vi "ReadCalibrationData.vi"(0 "reference in":refnum<class "BME280.lvclass">, 5 "error in (no error)":errorcluster, 6 "LINX Resource":T2={"IO"=enum."Remote", "Interface"=enum."Serial", "LINX Device Config"={"Interface"=enum."Serial", "COM Port"="COM13", "TCP Configuration"={"IP Address"="", "Port"=0}, "Device Family"=1, "Device ID"=1, "Device Name"="myRIO-1900", "TCP Ref"=refnum, "Channels"={"DI"=[0, 1, 2, 3, 4, 5, 6, 7, 8, 9, 10, 11, 12, 13, 14, 15, 16, 17, 18, 19, 20, 21, 22, 23, 24, 25, 26, 27, 28, 29, 30, 31, 32, 33, 34, 35, 36, 37, 38, 39, 40, 41, 42, 43, 44, 45, 46], "DO"=[0, 1, 2, 3, 4, 5, 6, 7, 8, 9, 10, 11, 12, 13, 14, 15, 16, 17, 18, 19, 20, 21, 22, 23, 24, 25, 26, 27, 28, 29, 30, 31, 32, 33, 34, 35, 36, 37, 38, 39, 40, 41, 42, 43, 44, 45, 46], "AI"=[0, 1, 2, 3, 4, 5, 6, 7, 8, 9, 10, 11], "AO"=[], "PWM"=[3, 5, 6, 9, 10], "QE"=[], "UART"=[0, 1], "I2C 2"=[0], "SPI"=[0], "CAN"=[], "Servo"=[], "AI Ref (V)"=0.0, "AI Resolution (Bits)"=0, "AO Ref (V)"=0.0, "AO Resolution (Bits)"=0}}}, 8 "I2C Channel (0)":u8=1) -> (12 "LINX Resource":T2={"IO"=enum."Remote", "Interface"=enum."Serial", "LINX Device Config"={"Interface"=enum."Serial", "COM Port"="COM13", "TCP Configuration"={"IP Address"="", "Port"=0}, "Device Family"=1, "Device ID"=1, "Device Name"="myRIO-1900", "TCP Ref"=refnum, "Channels"={"DI"=[0, 1, 2, 3, 4, 5, 6, 7, 8, 9, 10, 11, 12, 13, 14, 15, 16, 17, 18, 19, 20, 21, 22, 23, 24, 25, 26, 27, 28, 29, 30, 31, 32, 33, 34, 35, 36, 37, 38, 39, 40, 41, 42, 43, 44, 45, 46], "DO"=[0, 1, 2, 3, 4, 5, 6, 7, 8, 9, 10, 11, 12, 13, 14, 15, 16, 17, 18, 19, 20, 21, 22, 23, 24, 25, 26, 27, 28, 29, 30, 31, 32, 33, 34, 35, 36, 37, 38, 39, 40, 41, 42, 43, 44, 45, 46], "AI"=[0, 1, 2, 3, 4, 5, 6, 7, 8, 9, 10, 11], "AO"=[], "PWM"=[3, 5, 6, 9, 10], "QE"=[], "UART"=[0, 1], "I2C 2"=[0], "SPI"=[0], "CAN"=[], "Servo"=[], "AI Ref (V)"=0.0, "AI Resolution (Bits)"=0, "AO Ref (V)"=0.0, "AO Resolution (Bits)"=0}}}, 14 "reference out":refnum<class "BME280.lvclass">, 16 "TrimmingParameters":T1, 19 "error out":errorcluster)   [LabVIEW 2014, in "BME280.lvclass"]
uses:
  BME280.lvclass
  <vilib>/MakerHub/LINX/Private/Type Defs/LINX Ref.ctl
  <vilib>/MakerHub/LINX/Private/Type Defs/Platform.ctl
  <vilib>/MakerHub/LINX/Private/Type Defs/Interface.ctl
  <vilib>/MakerHub/LINX/Private/Device/Type Defs/LINX Device Config.ctl
  <vilib>/MakerHub/LINX/Private/Device/Type Defs/TCP Config.ctl
  <vilib>/MakerHub/LINX/Private/Device/Type Defs/Channels.ctl
  TrimmingParameters.ctl
  <vilib>/MakerHub/LINX/Private/Local IO/LinxI2cWrite.vi
  <vilib>/MakerHub/LINX/Public/Utilities/Check Channel.vi
  <vilib>/MakerHub/LINX/Private/Local IO/Handle Errors.vi
  <vilib>/MakerHub/LINX/Private/Utilties/Generate Error.vi
  <vilib>/MakerHub/LINX/LMH-LINX.lvlib
  <vilib>/MakerHub/LINX/Private/Device/Device.lvlib
panel:
  out "Data 3":u8[](array[numeric])
  out "Data 2":u8[](array[numeric])
  out "Data":u8[](array[numeric])
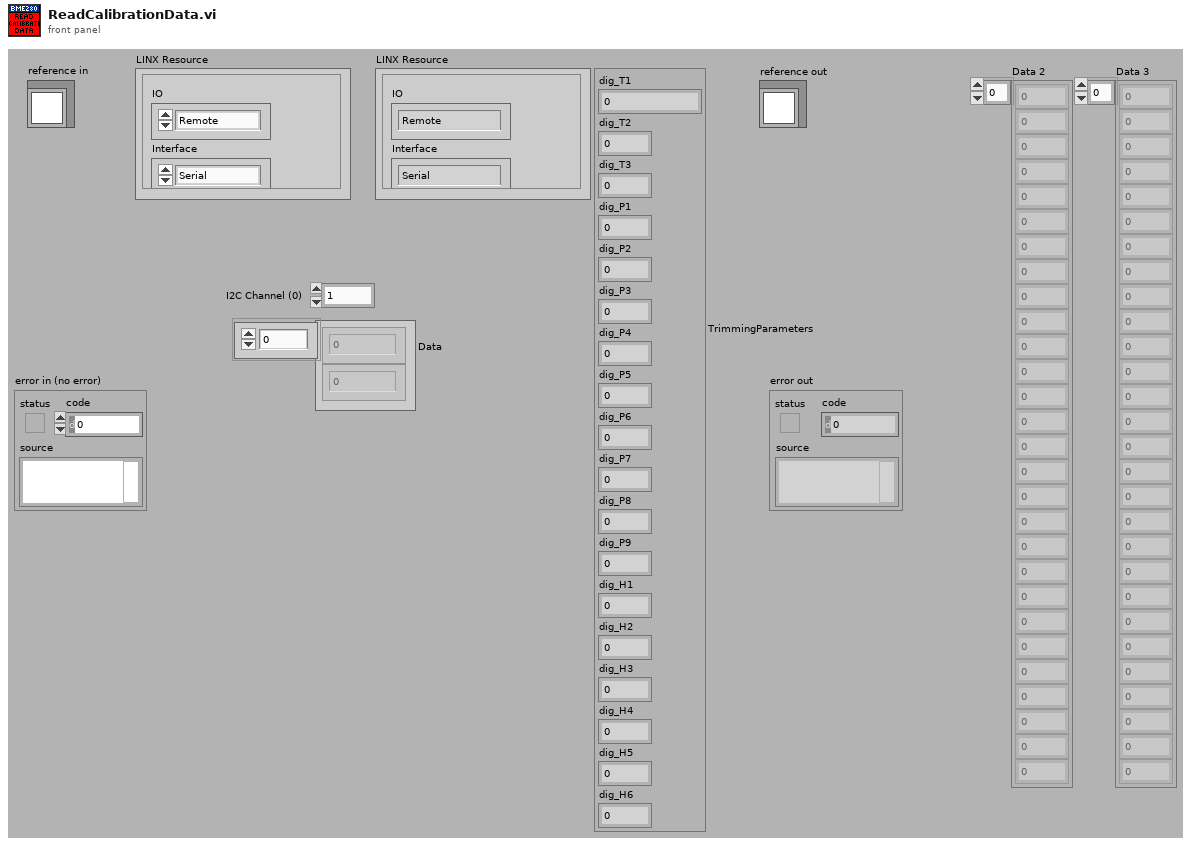
[diagram p1: front panel]
types:
  T1 = typedef "BME280.lvclass/TrimmingParameters.ctl" = cluster{"dig_T1":u16, "dig_T2":i16, "dig_T3":i16, "dig_P1":u16, "dig_P2":i16, "dig_P3":i16, "dig_P4":i16, "dig_P5":i16, "dig_P6":i16, "dig_P7":i16, "dig_P8":i16, "dig_P9":i16, "dig_H1":u8, "dig_H2":i16, "dig_H3":u8, "dig_H4":i16, "dig_H5":i16, "dig_H6":i8}
  T2 = typedef "LMH-LINX.lvlib/LINX Ref.ctl" = cluster{"IO":T3, "Interface":T4, "LINX Device Config":T5}
  T3 = typedef "LMH-LINX.lvlib/Platform.ctl" = enum16{"Remote", "Local"}
  T4 = typedef "LMH-LINX.lvlib/Interface.ctl" = enum16{"Serial", "TCP"}
  T5 = typedef "LMH-LINX.lvlib/Device.lvlib/LINX Device Config.ctl" = cluster{"Interface":T4, "COM Port":refnum<visa-resource-name>, "TCP Configuration":T6, "Device Family":u8, "Device ID":u8, "Device Name":string, "TCP Ref":refnum<k5>, "Channels":T7}
  T6 = typedef "LMH-LINX.lvlib/Device.lvlib/TCP Config.ctl" = cluster{"IP Address":string, "Port":u16}
  T7 = typedef "LMH-LINX.lvlib/Channels.ctl" = cluster{"DI":u8[], "DO":u8[], "AI":u8[], "AO":u8[], "PWM":u8[], "QE":u8[], "UART":u8[], "I2C 2":u8[], "SPI":u8[], "CAN":u8[], "Servo":u8[], "AI Ref (V)":dbl, "AI Resolution (Bits)":u8, "AO Ref (V)":dbl, "AO Resolution (Bits)":u8}
  T8 = typedef "BME280.lvclass/ObjectAttributes.ctl" = cluster{"I2C Slave Address":u8, "TrimmingParameters":T1, "t_fine":i32}
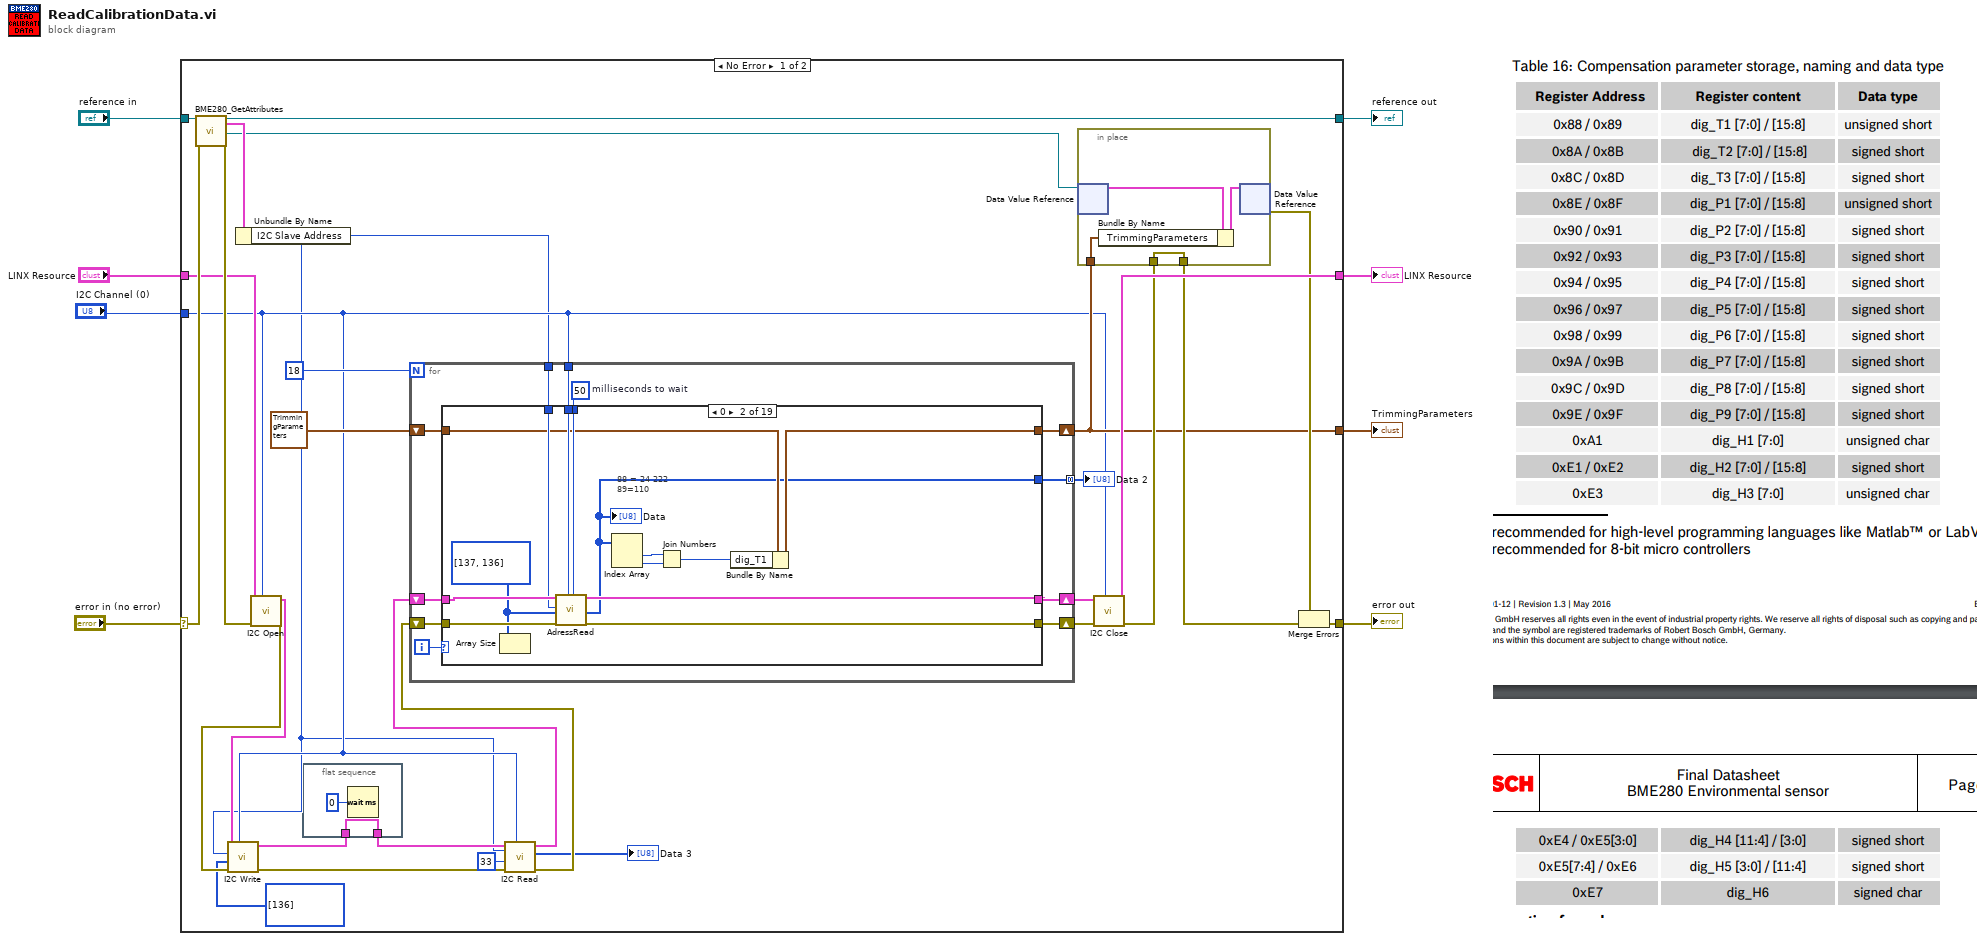
[diagram p0: block diagram]
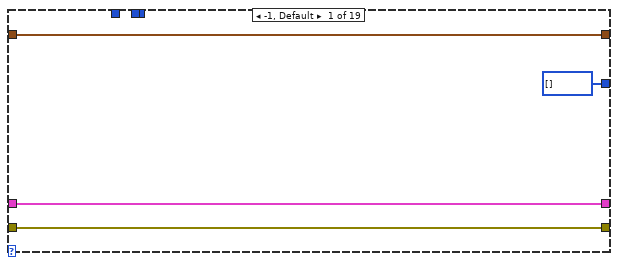
[diagram p2: hidden frame]
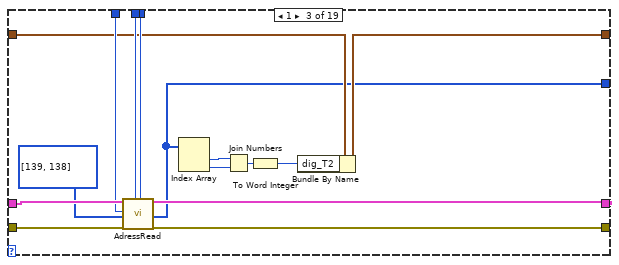
[diagram p3: hidden frame]
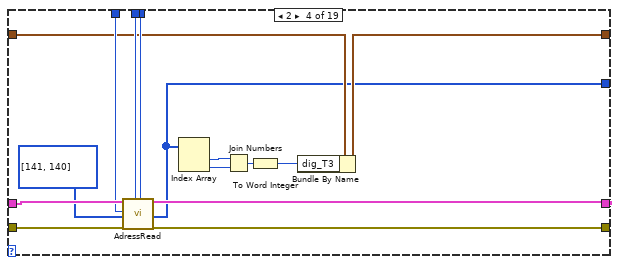
[diagram p4: hidden frame]
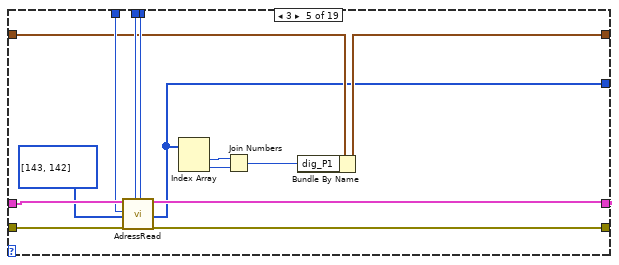
[diagram p5: hidden frame]
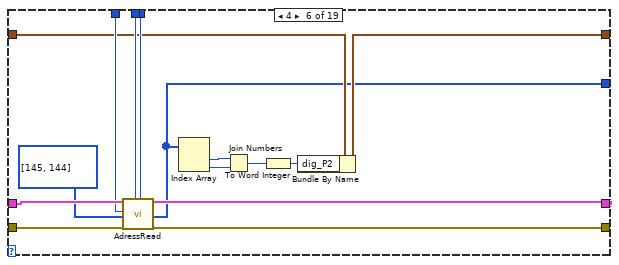
[diagram p6: hidden frame]
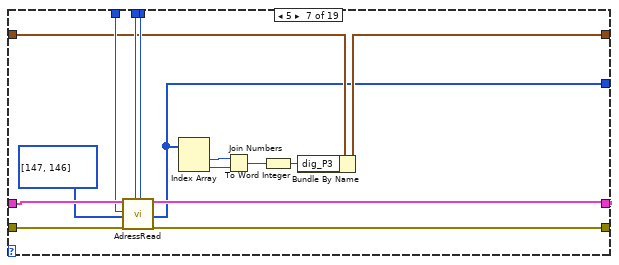
[diagram p7: hidden frame]
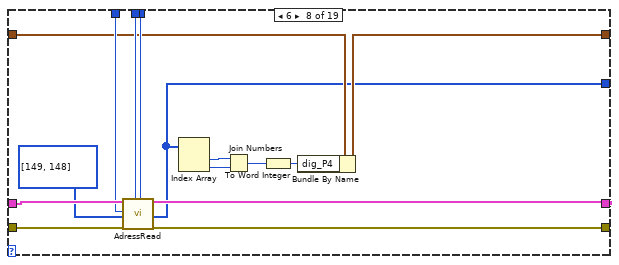
[diagram p8: hidden frame]
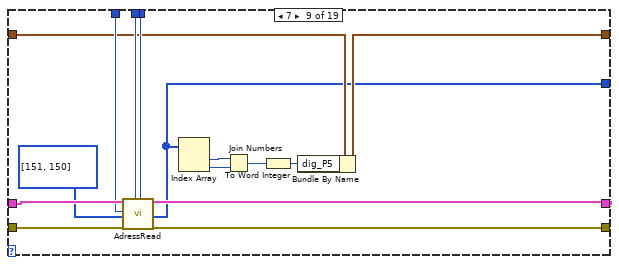
[diagram p9: hidden frame]
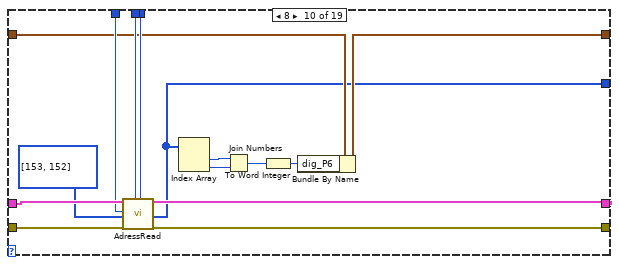
[diagram p10: hidden frame]
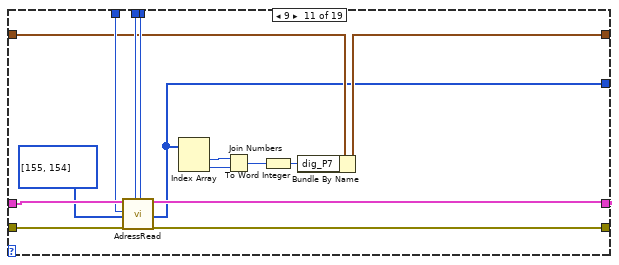
[diagram p11: hidden frame]
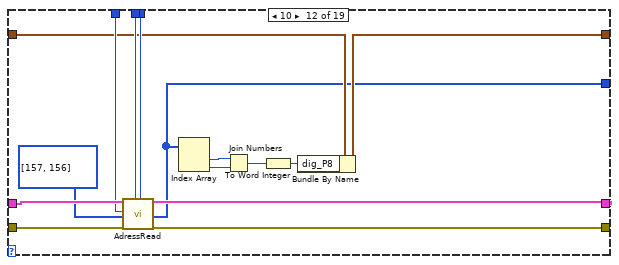
[diagram p12: hidden frame]
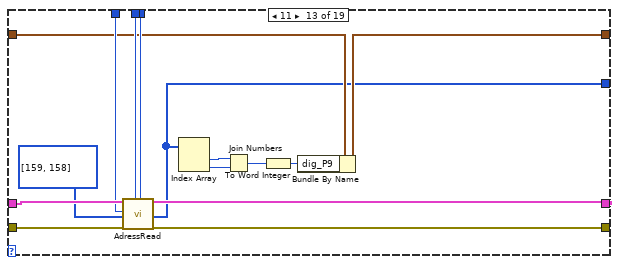
[diagram p13: hidden frame]
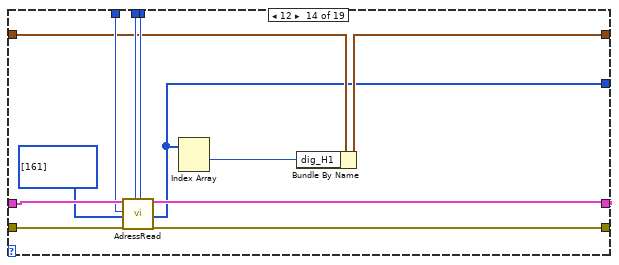
[diagram p14: hidden frame]
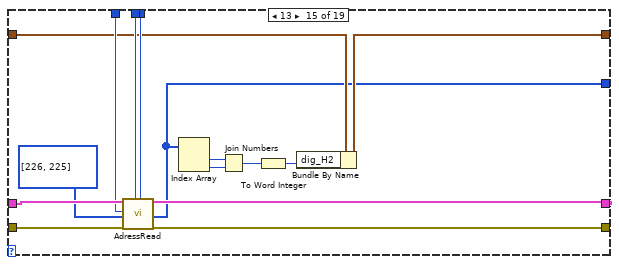
[diagram p15: hidden frame]
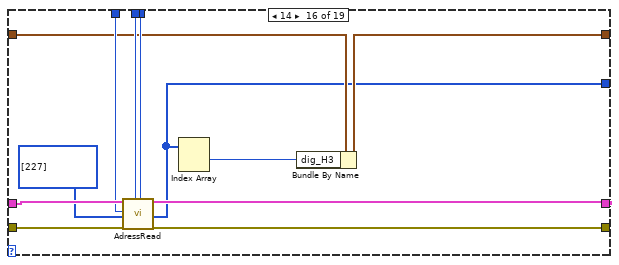
[diagram p16: hidden frame]
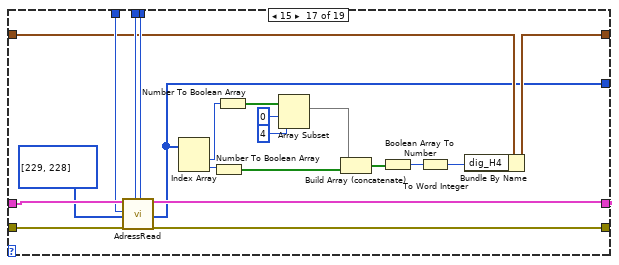
[diagram p17: hidden frame]
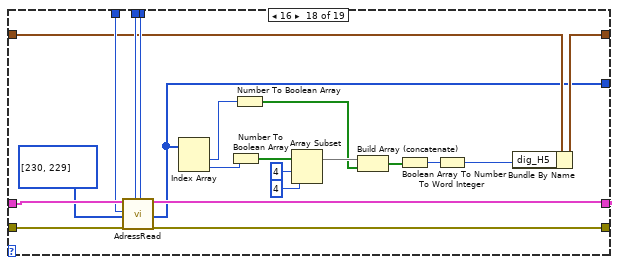
[diagram p18: hidden frame]
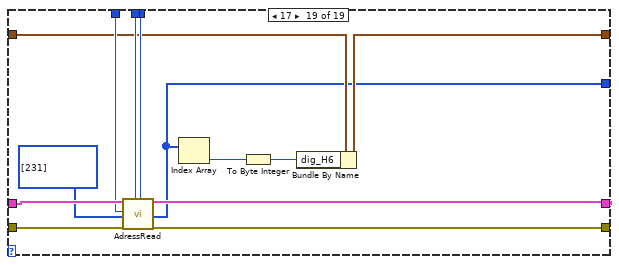
[diagram p19: hidden frame]
diagram:
  n1 = case shown="No Error" "error in (no error)" {
    selector: "error in (no error)" -> [w38 w334]
    tunnel: [w24 w334] -> w7
    tunnel: [w36 w333] -> w5
    tunnel: "reference in" -> [w37 w333]
    tunnel: "LINX Resource" -> [w34 w332]
    tunnel: [w33 w332] -> w3
    tunnel: "I2C Channel (0)" -> [w13 _]
    tunnel: [w22 _] -> w1
    frame No Error {
      n2 = call "BME280_GetAttributes.vi"("reference in"=w37, "error in (no error)"=w38) -> ("reference out"=w36:refnum<class "BME280.lvclass">, "Data"=w32:T8, "DataRef"=w26:refnum<data-value>, "error out"=w35:errorcluster)  [unwired: 14 in]
      n3 = Unbundle By Name(w32) -> ("I2C Slave Address"=w12:u8)
      n4 = call <vilib>:"I2C Open.vi"("I2C Channel (0)"=w13, "Error In"=w35, "LINX Resource"=w34) -> ("Error Out"=w15:errorcluster, "LINX Resource"=w17:T2)  [unwired: 7 in]
      n5 = call <vilib>:"I2C Write.vi"("I2C Channel"=w13, "Error In"=w15, "Data"=u8[] [136] ("Adress"), "I2C Slave Address (0)"=w12, "LINX Resource"=w17) -> ("Error Out"=w18:errorcluster, "LINX Resource"=w19:T2)  [unwired: 5 in]
      n6 = flat-sequence {
        tunnel: [w40] -> w20
        tunnel: w19 -> [w40]
        frame #0 {
          n7 = Wait (ms)(milliseconds to wait=u32 0) -> ()  [unwired: 1 out]
        }
      }
      n8 = call <vilib>:"I2C Read.vi"("I2C Channel"=w13, "Error In"=w18, "Bytes To Read"=u8 33, "I2C Slave Address (0)"=w12, "LINX Resource"=w20) -> ("Error Out"=w14:errorcluster, "Data"=→"Data 3":u8[], "LINX Resource"=w16:T2)  [unwired: 4 in]
      n9 = for {
        N: 18 -> [_]
        shift-right: [w50] -> w31
        shift-left: w16 -> [w51]
        shift-right: [w48] -> w30
        shift-left: w14 -> [w49]
        shift-right: [w44] -> w22
        shift-left: T1 {"dig_T1"=0, "dig_T2"=0, "dig_T3"=0, "dig_P1"=0, "dig_P2"=0, "dig_P3"=0, "dig_P4"=0, "dig_P5"=0, "dig_P6"=0, "dig_P7"=0, "dig_P8"=0, "dig_P9"=0, "dig_H1"=0, "dig_H2"=0, "dig_H3"=0, "dig_H4"=0, "dig_H5"=0, "dig_H6"=0} ("TrimmingParameters") -> [w45]
        tunnel: w12 -> [w43]
        tunnel: w13 -> [w42]
        tunnel: [w41] -> w21 mode=concatenating
        i -> [w46]
        w47 = u32 50  # milliseconds to wait
        n10 = case shown="0" w46 {
          tunnel: w51 -> [w55 w66 w81 w96 w110 w125 w140 w155 w170 w185 w200 w215 w230 w242 w257 w269 w290 w311 w324]
          tunnel: [w55 w69 w84 w99 w113 w128 w143 w158 w173 w188 w203 w218 w233 w245 w260 w272 w293 w314 w327] -> w50
          tunnel: w49 -> [w54 w68 w83 w98 w112 w127 w142 w157 w172 w187 w202 w217 w232 w244 w259 w271 w292 w313 w326]
          tunnel: [w54 w67 w82 w97 w111 w126 w141 w156 w171 w186 w201 w216 w231 w243 w258 w270 w291 w312 w325] -> w48
          tunnel: w47 -> [_ w65 w79 w94 w108 w123 w138 w153 w168 w183 w198 w213 w228 w240 w255 w267 w288 w309 w322]
          tunnel: w45 -> [w53 w60 w74 w89 w103 w118 w133 w148 w163 w178 w193 w208 w223 w237 w252 w264 w285 w306 w319]
          tunnel: [w53 w59 w73 w88 w102 w117 w132 w147 w162 w177 w192 w207 w222 w236 w251 w263 w284 w305 w318] -> w44
          tunnel: w43 -> [_ w63 w77 w92 w106 w121 w136 w151 w166 w181 w196 w211 w226 w238 w253 w265 w286 w307 w320]
          tunnel: w42 -> [_ w64 w78 w93 w107 w122 w137 w152 w167 w182 w197 w212 w227 w239 w254 w266 w287 w308 w321]
          tunnel: [u8[] [] ("Data") w56 w70 w85 w100 w114 w129 w144 w159 w174 w189 w204 w219 w234 w246 w261 w273 w294 w315] -> w41
          frame -1, Default {
          }
          frame 0 {
            w57 = u8[] [137, 136] ("Adress")
            # "88 = 24 222\n89=110"
            n11 = Array Size(array=w57) -> ()  [unwired: 1 out]
            n12 = call "AdressRead.vi"("LINX Resource in"=w66, "I2C Slave Address"=w63, "Adress"=w57, "error in (no error)"=w68, "I2C Channel"=w64, "milliseconds to wait"=w65) -> ("LINX Resource out"=w69:T2, "Data"=w56:u8[], "error out"=w67:errorcluster)  [unwired: 11 in]
            "Data" <- w56
            n13 = Index Array(array=w56) -> (element #1=w62:u8, element #2=w61:u8)  [unwired: 2 in]
            n14 = Join Numbers(hi=w62, lo=w61) -> ((hi.lo)=w58:u16)
            n15 = Bundle By Name(cluster=w60, "dig_T1"=w58) -> (w59:T1)
          }
          frame 1 {
            n16 = call "AdressRead.vi"("LINX Resource in"=w81, "I2C Slave Address"=w77, "Adress"=u8[] [139, 138], "error in (no error)"=w83, "I2C Channel"=w78, "milliseconds to wait"=w79) -> ("LINX Resource out"=w84:T2, "Data"=w70:u8[], "error out"=w82:errorcluster)  [unwired: 11 in]
            n17 = Index Array(array=w70) -> (element #1=w76:u8, element #2=w75:u8)  [unwired: 2 in]
            n18 = Join Numbers(hi=w76, lo=w75) -> ((hi.lo)=w72:u16)
            n19 = To Word Integer(number=w72) -> (16bit integer=w71:i16)
            n20 = Bundle By Name(cluster=w74, "dig_T2"=w71) -> (w73:T1)
          }
          frame 2 {
            n21 = call "AdressRead.vi"("LINX Resource in"=w96, "I2C Slave Address"=w92, "Adress"=u8[] [141, 140], "error in (no error)"=w98, "I2C Channel"=w93, "milliseconds to wait"=w94) -> ("LINX Resource out"=w99:T2, "Data"=w85:u8[], "error out"=w97:errorcluster)  [unwired: 11 in]
            n22 = Index Array(array=w85) -> (element #1=w91:u8, element #2=w90:u8)  [unwired: 2 in]
            n23 = Join Numbers(hi=w91, lo=w90) -> ((hi.lo)=w87:u16)
            n24 = To Word Integer(number=w87) -> (16bit integer=w86:i16)
            n25 = Bundle By Name(cluster=w89, "dig_T3"=w86) -> (w88:T1)
          }
          frame 3 {
            n26 = call "AdressRead.vi"("LINX Resource in"=w110, "I2C Slave Address"=w106, "Adress"=u8[] [143, 142], "error in (no error)"=w112, "I2C Channel"=w107, "milliseconds to wait"=w108) -> ("LINX Resource out"=w113:T2, "Data"=w100:u8[], "error out"=w111:errorcluster)  [unwired: 11 in]
            n27 = Index Array(array=w100) -> (element #1=w105:u8, element #2=w104:u8)  [unwired: 2 in]
            n28 = Join Numbers(hi=w105, lo=w104) -> ((hi.lo)=w101:u16)
            n29 = Bundle By Name(cluster=w103, "dig_P1"=w101) -> (w102:T1)
          }
          frame 4 {
            n30 = call "AdressRead.vi"("LINX Resource in"=w125, "I2C Slave Address"=w121, "Adress"=u8[] [145, 144], "error in (no error)"=w127, "I2C Channel"=w122, "milliseconds to wait"=w123) -> ("LINX Resource out"=w128:T2, "Data"=w114:u8[], "error out"=w126:errorcluster)  [unwired: 11 in]
            n31 = Index Array(array=w114) -> (element #1=w120:u8, element #2=w119:u8)  [unwired: 2 in]
            n32 = Join Numbers(hi=w120, lo=w119) -> ((hi.lo)=w116:u16)
            n33 = To Word Integer(number=w116) -> (16bit integer=w115:i16)
            n34 = Bundle By Name(cluster=w118, "dig_P2"=w115) -> (w117:T1)
          }
          frame 5 {
            n35 = call "AdressRead.vi"("LINX Resource in"=w140, "I2C Slave Address"=w136, "Adress"=u8[] [147, 146], "error in (no error)"=w142, "I2C Channel"=w137, "milliseconds to wait"=w138) -> ("LINX Resource out"=w143:T2, "Data"=w129:u8[], "error out"=w141:errorcluster)  [unwired: 11 in]
            n36 = Index Array(array=w129) -> (element #1=w135:u8, element #2=w134:u8)  [unwired: 2 in]
            n37 = Join Numbers(hi=w135, lo=w134) -> ((hi.lo)=w131:u16)
            n38 = To Word Integer(number=w131) -> (16bit integer=w130:i16)
            n39 = Bundle By Name(cluster=w133, "dig_P3"=w130) -> (w132:T1)
          }
          frame 6 {
            n40 = call "AdressRead.vi"("LINX Resource in"=w155, "I2C Slave Address"=w151, "Adress"=u8[] [149, 148], "error in (no error)"=w157, "I2C Channel"=w152, "milliseconds to wait"=w153) -> ("LINX Resource out"=w158:T2, "Data"=w144:u8[], "error out"=w156:errorcluster)  [unwired: 11 in]
            n41 = Index Array(array=w144) -> (element #1=w150:u8, element #2=w149:u8)  [unwired: 2 in]
            n42 = Join Numbers(hi=w150, lo=w149) -> ((hi.lo)=w146:u16)
            n43 = To Word Integer(number=w146) -> (16bit integer=w145:i16)
            n44 = Bundle By Name(cluster=w148, "dig_P4"=w145) -> (w147:T1)
          }
          frame 7 {
            n45 = call "AdressRead.vi"("LINX Resource in"=w170, "I2C Slave Address"=w166, "Adress"=u8[] [151, 150], "error in (no error)"=w172, "I2C Channel"=w167, "milliseconds to wait"=w168) -> ("LINX Resource out"=w173:T2, "Data"=w159:u8[], "error out"=w171:errorcluster)  [unwired: 11 in]
            n46 = Index Array(array=w159) -> (element #1=w165:u8, element #2=w164:u8)  [unwired: 2 in]
            n47 = Join Numbers(hi=w165, lo=w164) -> ((hi.lo)=w161:u16)
            n48 = To Word Integer(number=w161) -> (16bit integer=w160:i16)
            n49 = Bundle By Name(cluster=w163, "dig_P5"=w160) -> (w162:T1)
          }
          frame 8 {
            n50 = call "AdressRead.vi"("LINX Resource in"=w185, "I2C Slave Address"=w181, "Adress"=u8[] [153, 152], "error in (no error)"=w187, "I2C Channel"=w182, "milliseconds to wait"=w183) -> ("LINX Resource out"=w188:T2, "Data"=w174:u8[], "error out"=w186:errorcluster)  [unwired: 11 in]
            n51 = Index Array(array=w174) -> (element #1=w180:u8, element #2=w179:u8)  [unwired: 2 in]
            n52 = Join Numbers(hi=w180, lo=w179) -> ((hi.lo)=w176:u16)
            n53 = To Word Integer(number=w176) -> (16bit integer=w175:i16)
            n54 = Bundle By Name(cluster=w178, "dig_P6"=w175) -> (w177:T1)
          }
          frame 9 {
            n55 = call "AdressRead.vi"("LINX Resource in"=w200, "I2C Slave Address"=w196, "Adress"=u8[] [155, 154], "error in (no error)"=w202, "I2C Channel"=w197, "milliseconds to wait"=w198) -> ("LINX Resource out"=w203:T2, "Data"=w189:u8[], "error out"=w201:errorcluster)  [unwired: 11 in]
            n56 = Index Array(array=w189) -> (element #1=w195:u8, element #2=w194:u8)  [unwired: 2 in]
            n57 = Join Numbers(hi=w195, lo=w194) -> ((hi.lo)=w191:u16)
            n58 = To Word Integer(number=w191) -> (16bit integer=w190:i16)
            n59 = Bundle By Name(cluster=w193, "dig_P7"=w190) -> (w192:T1)
          }
          frame 10 {
            n60 = call "AdressRead.vi"("LINX Resource in"=w215, "I2C Slave Address"=w211, "Adress"=u8[] [157, 156], "error in (no error)"=w217, "I2C Channel"=w212, "milliseconds to wait"=w213) -> ("LINX Resource out"=w218:T2, "Data"=w204:u8[], "error out"=w216:errorcluster)  [unwired: 11 in]
            n61 = Index Array(array=w204) -> (element #1=w210:u8, element #2=w209:u8)  [unwired: 2 in]
            n62 = Join Numbers(hi=w210, lo=w209) -> ((hi.lo)=w206:u16)
            n63 = To Word Integer(number=w206) -> (16bit integer=w205:i16)
            n64 = Bundle By Name(cluster=w208, "dig_P8"=w205) -> (w207:T1)
          }
          frame 11 {
            n65 = call "AdressRead.vi"("LINX Resource in"=w230, "I2C Slave Address"=w226, "Adress"=u8[] [159, 158], "error in (no error)"=w232, "I2C Channel"=w227, "milliseconds to wait"=w228) -> ("LINX Resource out"=w233:T2, "Data"=w219:u8[], "error out"=w231:errorcluster)  [unwired: 11 in]
            n66 = Index Array(array=w219) -> (element #1=w225:u8, element #2=w224:u8)  [unwired: 2 in]
            n67 = Join Numbers(hi=w225, lo=w224) -> ((hi.lo)=w221:u16)
            n68 = To Word Integer(number=w221) -> (16bit integer=w220:i16)
            n69 = Bundle By Name(cluster=w223, "dig_P9"=w220) -> (w222:T1)
          }
          frame 12 {
            n70 = call "AdressRead.vi"("LINX Resource in"=w242, "I2C Slave Address"=w238, "Adress"=u8[] [161], "error in (no error)"=w244, "I2C Channel"=w239, "milliseconds to wait"=w240) -> ("LINX Resource out"=w245:T2, "Data"=w234:u8[], "error out"=w243:errorcluster)  [unwired: 11 in]
            n71 = Index Array(array=w234) -> (element #1=w235:u8)  [unwired: 2 in, 1 out]
            n72 = Bundle By Name(cluster=w237, "dig_H1"=w235) -> (w236:T1)
          }
          frame 13 {
            n73 = call "AdressRead.vi"("LINX Resource in"=w257, "I2C Slave Address"=w253, "Adress"=u8[] [226, 225], "error in (no error)"=w259, "I2C Channel"=w254, "milliseconds to wait"=w255) -> ("LINX Resource out"=w260:T2, "Data"=w246:u8[], "error out"=w258:errorcluster)  [unwired: 11 in]
            n74 = Index Array(array=w246) -> (element #1=w249:u8, element #2=w248:u8)  [unwired: 2 in]
            n75 = Join Numbers(hi=w249, lo=w248) -> ((hi.lo)=w250:u16)
            n76 = To Word Integer(number=w250) -> (16bit integer=w247:i16)
            n77 = Bundle By Name(cluster=w252, "dig_H2"=w247) -> (w251:T1)
          }
          frame 14 {
            n78 = call "AdressRead.vi"("LINX Resource in"=w269, "I2C Slave Address"=w265, "Adress"=u8[] [227], "error in (no error)"=w271, "I2C Channel"=w266, "milliseconds to wait"=w267) -> ("LINX Resource out"=w272:T2, "Data"=w261:u8[], "error out"=w270:errorcluster)  [unwired: 11 in]
            n79 = Index Array(array=w261) -> (element #1=w262:u8)  [unwired: 2 in, 1 out]
            n80 = Bundle By Name(cluster=w264, "dig_H3"=w262) -> (w263:T1)
          }
          frame 15 {
            n81 = call "AdressRead.vi"("LINX Resource in"=w290, "I2C Slave Address"=w286, "Adress"=u8[] [229, 228], "error in (no error)"=w292, "I2C Channel"=w287, "milliseconds to wait"=w288) -> ("LINX Resource out"=w293:T2, "Data"=w273:u8[], "error out"=w291:errorcluster)  [unwired: 11 in]
            n82 = Index Array(array=w273) -> (element #1=w282:u8, element #2=w283:u8)  [unwired: 2 in]
            n83 = Number To Boolean Array(number=w283) -> (Boolean array=w277:bool[])
            n84 = Number To Boolean Array(number=w282) -> (Boolean array=w281:bool[])
            n85 = Array Subset(array=w281, index=0, length=4) -> (w278:bool[])
            n86 = Build Array (concatenate)(w278, w277) -> (w276:bool[])
            n87 = Boolean Array To Number(Boolean array=w276) -> (number=w275:u32)
            n88 = To Word Integer(number=w275) -> (16bit integer=w274:i16)
            n89 = Bundle By Name(cluster=w285, "dig_H4"=w274) -> (w284:T1)
          }
          frame 16 {
            n90 = call "AdressRead.vi"("LINX Resource in"=w311, "I2C Slave Address"=w307, "Adress"=u8[] [230, 229], "error in (no error)"=w313, "I2C Channel"=w308, "milliseconds to wait"=w309) -> ("LINX Resource out"=w314:T2, "Data"=w294:u8[], "error out"=w312:errorcluster)  [unwired: 11 in]
            n91 = Index Array(array=w294) -> (element #1=w299:u8, element #2=w300:u8)  [unwired: 2 in]
            n92 = Number To Boolean Array(number=w300) -> (Boolean array=w298:bool[])
            n93 = Number To Boolean Array(number=w299) -> (Boolean array=w296:bool[])
            n94 = Array Subset(array=w298, index=4, length=4) -> (w297:bool[])
            n95 = Build Array (concatenate)(w297, w296) -> (w302:bool[])
            n96 = Boolean Array To Number(Boolean array=w302) -> (number=w301:u32)
            n97 = To Word Integer(number=w301) -> (16bit integer=w295:i16)
            n98 = Bundle By Name(cluster=w306, "dig_H5"=w295) -> (w305:T1)
          }
          frame 17 {
            n99 = call "AdressRead.vi"("LINX Resource in"=w324, "I2C Slave Address"=w320, "Adress"=u8[] [231], "error in (no error)"=w326, "I2C Channel"=w321, "milliseconds to wait"=w322) -> ("LINX Resource out"=w327:T2, "Data"=w315:u8[], "error out"=w325:errorcluster)  [unwired: 11 in]
            n100 = Index Array(array=w315) -> (element=w317:u8)  [unwired: 1 in]
            n101 = To Byte Integer(number=w317) -> (8bit integer=w316:i8)
            n102 = Bundle By Name(cluster=w319, "dig_H6"=w316) -> (w318:T1)
          }
        }
      }
      "Data 2" <- w21
      n103 = call <vilib>:"I2C Close.vi"("I2C Channel (0)"=w13, "Error In"=w30, "LINX Resource"=w31) -> ("Error Out"=w25:errorcluster, "LINX Resource"=w33:T2)  [unwired: 7 in]
      n104 = in-place {
        in-place-border: w22 -> [w329]
        in-place-border: [w328] -> w23
        in-place-border: w25 -> [w328]
        n105 = in-place-dvr #1(w26) -> (w331:T8)  [unwired: 1 out]
        n106 = Bundle By Name(cluster=w331, "TrimmingParameters"=w329) -> (w330:T8)
        n107 = in-place-dvr #1(w330) -> (w27:errorcluster)  [unwired: 1 out]
      }
      n108 = Merge Errors(w27, w23) -> (w24:errorcluster)
    }
    frame Error {
    }
  }
  "error out" <- w7
  "reference out" <- w5
  "LINX Resource" <- w3
  "TrimmingParameters" <- w1
